vi "Find Implemented Msgs.vi"(10 "Path":path) -> (2 "Implemented Msgs":T1)   [LabVIEW 2020, in "jettl.lvlib" / "Actor.lvlib" / "Base Actor.lvclass"]
uses:
  Base Actor.lvclass
  Implemented Msgs.ctl
  Msg/Msg.lvclass
  Actor/Actor.lvclass
  Actor.lvlib
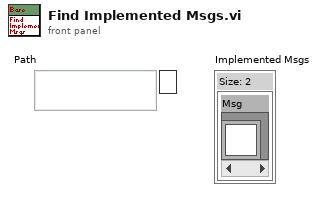
[diagram p1: front panel]
types:
  T1 = typedef "jettl.lvlib/Actor.lvlib/Implemented Msgs.ctl" = set{refnum<class "Msg.lvclass">}
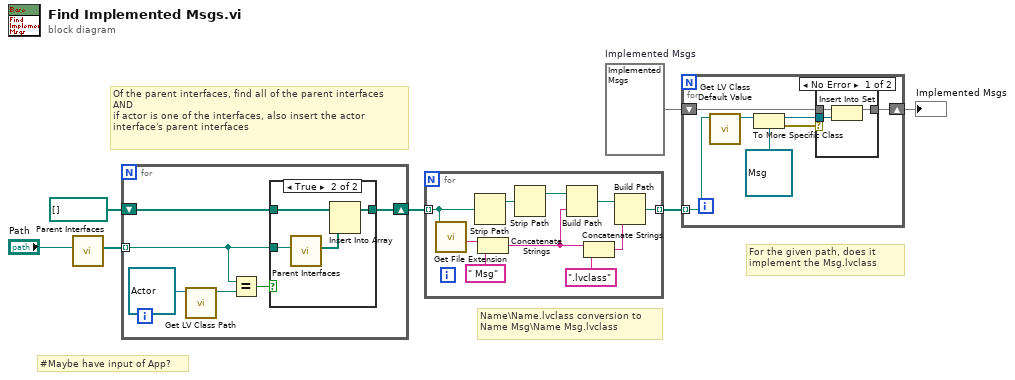
[diagram p0: block diagram]
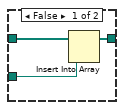
[diagram p2: hidden frame]
diagram:
  w4 = T1 {}  # Implemented Msgs
  # "#Maybe have input of App?"
  # "For the given path, does it implement the Msg.lvclass"
  # "Name\\Name.lvclass conversion to\nName Msg\\Name Msg.lvclass"
  # "Of the parent interfaces, find all of the parent interfaces\nAND\nif actor is one of the interfaces, also insert the actor interface's parent interfaces"
  n1 = call "Parent Interfaces.vi"("Path"="Path") -> ("Parent Interface Paths"=w7:path[])  [unwired: 9 in, 1 out]
  n2 = for {
    tunnel: w7 -> [w9] mode=indexing
    shift-right: [w11] -> w5
    shift-left: path[] [] ("Array 2") -> [w10]
    n3 = call <vilib>:"Get LV Class Path.vi"("object"=refnum<class "Actor.lvclass"> refnum ("jettl.lvlib:Actor.lvlib:Actor.lvclass")) -> ("class path"=w8:path)  [unwired: 9 in, 1 out]
    n4 = Equal?(x=w9, y=w8) -> (x = y?=w12:bool)
    n5 = case shown="True" w12 {
      tunnel: w9 -> [w14 w17]
      tunnel: [w15 w19] -> w11
      tunnel: w10 -> [w16 w20]
      frame False {
        n6 = Insert Into Array(array=w16, new element=w14) -> (w15:path[])  [unwired: 1 in]
      }
      frame True {
        n7 = call "Parent Interfaces.vi"("Path"=w17) -> ("Parent Interface Paths"=w18:path[])  [unwired: 9 in, 1 out]
        n8 = Insert Into Array(array=w20, new element=w18) -> (w19:path[])  [unwired: 1 in]
      }
    }
  }
  n9 = for {
    tunnel: w5 -> [w30] mode=indexing
    tunnel: [w26] -> w3 mode=indexing
    n10 = call <vilib>:"Get File Extension.vi"("file"=w30) -> ("filename without extension"=w22:string)  [unwired: 6 in, 4 out]
    n11 = Strip Path(path=w30) -> (stripped path=w29:path)  [unwired: 1 out]
    n12 = Concatenate Strings(w22, " Msg" ("string")) -> (w21:string)
    n13 = Strip Path(path=w29) -> (stripped path=w24:path)  [unwired: 1 out]
    n14 = Build Path(base path=w24, name or relative path=w21) -> (appended path=w23:path)
    n15 = Concatenate Strings(w21, ".lvclass" ("string")) -> (w28:string)
    n16 = Build Path(base path=w23, name or relative path=w28) -> (appended path=w26:path)
  }
  n17 = for {
    shift-right: [w36] -> w1
    shift-left: w4 -> [w37]
    tunnel: w3 -> [w33] mode=indexing
    n18 = call <vilib>:"Get LV Class Default Value.vi"("class path"=w33) -> ("object"=w34:refnum<class>)  [unwired: 9 in, 1 out]
    n19 = To More Specific Class(target class=refnum<class "Msg.lvclass"> refnum ("Msg"), reference=w34) -> (specific class reference=w35:refnum<class "Msg.lvclass">, error out=w31:errorcluster)  [unwired: 1 in]
    n20 = case shown="No Error" w31 {
      tunnel: w37 -> [w40 w41]
      tunnel: [w39 w41] -> w36
      tunnel: w35 -> [w38 _]
      frame No Error {
        n21 = Insert Into Set(10:w38, 11:w40) -> (3:w39:T1)  [unwired: 1 out]
      }
      frame Error {
      }
    }
  }
  "Implemented Msgs" <- w1
